vi "Get Localized Phrase Compact Interface 1D.vi"(1 "Key":string[](array[string])) -> (0 "Translated Phrase":string[](array[string]))   [LabVIEW 2020]
uses:
  Localization FGV Action -- Enum.ctl
panel:
  out "error_out":errorcluster
  in  "error_in":errorcluster
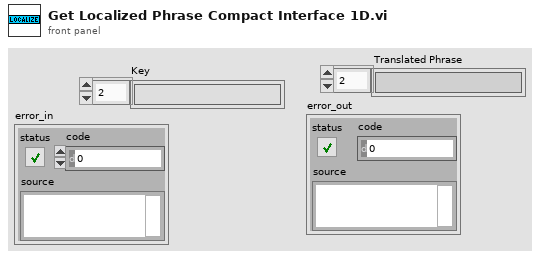
[diagram p1: front panel]
types:
  T1 = typedef "Localization FGV Action -- Enum.ctl" = enum16{"Read Dictionary", "Translate VIs", "Register VI", "Get Languages", "Translate Phrase", "Get Key For Phrase", "Get Phrase For Phrase", "Translate VI", "Unregister"}
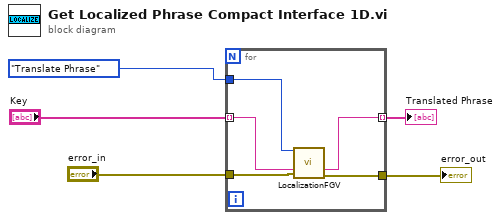
[diagram p0: block diagram]
diagram:
  n1 = for {
    tunnel: Localization_FGV_Action_--_Enum."Translate Phrase" ("Action") -> [w10]
    tunnel: "Key" -> [w9] mode=indexing
    tunnel: [w8] -> w3 mode=indexing
    tunnel: "error_in" -> [w7]
    tunnel: [w6] -> w1
    n2 = call "LocalizationFGV.vi"("Action"=w10, "Input"=w9, "error in"=w7) -> ("Result"=w8:string, "error out"=w6:errorcluster)  [unwired: 7 in, 4 out]
  }
  "Translated Phrase" <- w3
  "error_out" <- w1
